vi "Display_OriginalLoc_Coordinates.vi"(0 "Image In":T1(plugin-control), 1 "x":i32, 2 "y":i32, 5 "error in (no error)":errorcluster) -> (14 "Image Out":T1(plugin-control), 19 "error out":errorcluster)   [LabVIEW 2020]
doc: "Plots the location of the book in the map, using the generated coordinates as inputs."
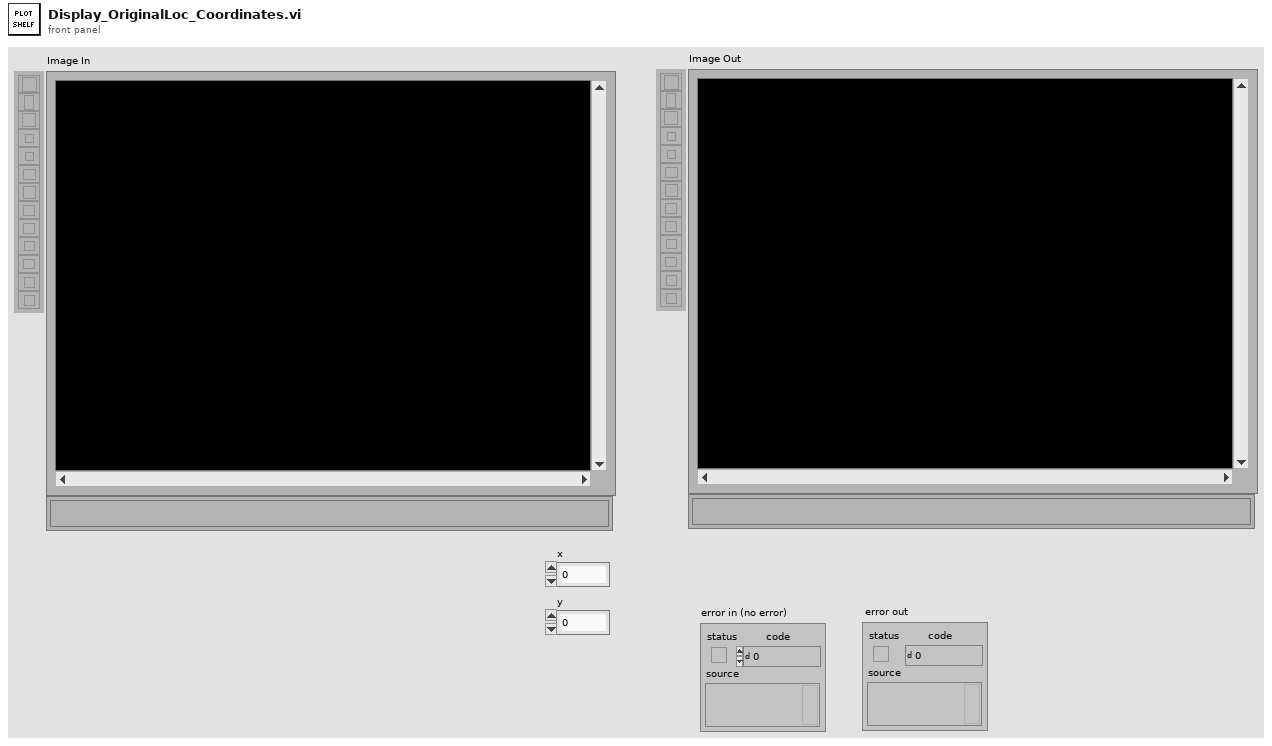
[diagram p1: front panel]
types:
  T1 = typedef "IMAQ Image.ctl" = refnum<image>
  T2 = typedef "IMAQ Rectangle" = cluster{"Left":i32, "Top":i32, "Right":i32, "Bottom":i32, "Rotation":dbl}
  T3 = typedef "ROI Descriptor" = cluster{"Global Rectangle":i32[], "Contours":cluster{"ID":enum32{"External", "Internal"}, "Type":u32, "Coordinates":i32[]}[]}
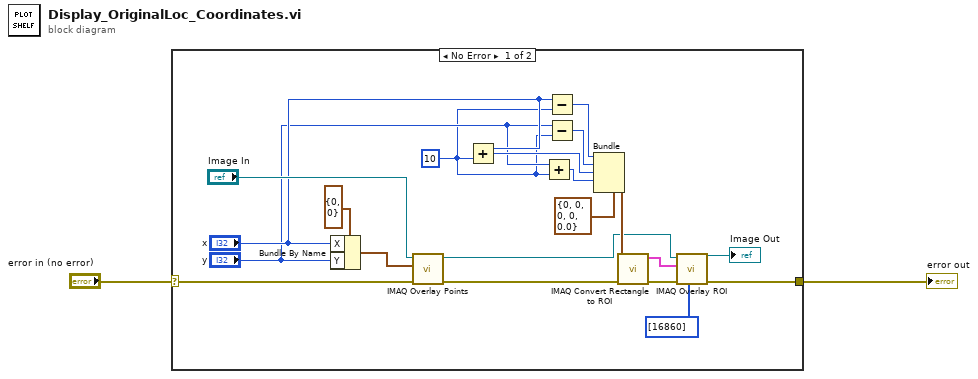
[diagram p0: block diagram]
diagram:
  n1 = case shown="No Error" "error in (no error)" {
    selector: "error in (no error)" -> [w4 w23]
    tunnel: [w11 w23] -> w2
    frame No Error {
      w5 = 10 ("y")
      n2 = Bundle By Name(cluster=cluster{"X":i32, "Y":i32} {"X"=0, "Y"=0} ("Point"), "X"="x", "Y"="y") -> (w21:cluster{"X":i32, "Y":i32})
      n3 = call "IMAQ Overlay Points"("error in (no error)"=w4, "Point"=w21, "Image"="Image In") -> ("error out"=w13:errorcluster, "Image Out"=w14:T1)  [unwired: 7 in]
      n4 = Add(x="x", y=w5) -> (x+y=w19:i32)
      n5 = Add(x="y", y=w5) -> (x+y=w18:i32)
      n6 = Subtract(x="x", y=w5) -> (x-y=w8:i32)
      n7 = Subtract(x="y", y=w5) -> (x-y=w6:i32)
      n8 = Bundle(cluster=T2 {"Left"=0, "Top"=0, "Right"=0, "Bottom"=0, "Rotation"=0.0} ("Rectangle"), "Left"=w8, "Top"=w6, "Right"=w19, "Bottom"=w18) -> (w15:T2)  [unwired: 1 in]
      n9 = call "IMAQ Convert Rectangle to ROI"("error in (no error)"=w13, "Rectangle"=w15) -> ("error out"=w12:errorcluster, "ROI Descriptor"=w16:T3)  [unwired: 7 in]
      n10 = call "IMAQ Overlay ROI"("Colors (Green)"=u32[] [16860], "error in (no error)"=w12, "ROI Descriptor"=w16, "Image"=w14) -> ("error out"=w11:errorcluster, "Image Out"=→"Image Out":T1)  [unwired: 6 in]
    }
    frame Error {
    }
  }
  "error out" <- w2
